vi "TDC_setHistogramParams.vi"(8 "Error In":errorcluster, 10 "Bin Count":i32, 11 "Bin Width":i32) -> (0 "Error Out":errorcluster)   [LabVIEW 2011]
uses:
  tdcbase.dll
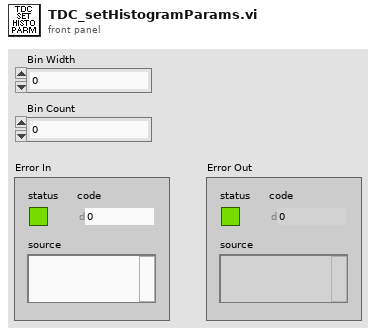
[diagram p1: front panel]
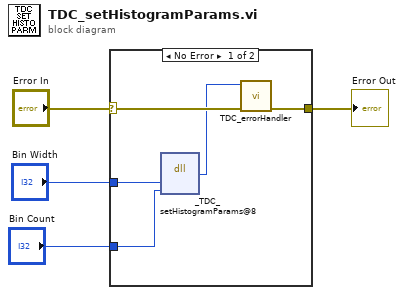
[diagram p0: block diagram]
diagram:
  n1 = case shown="No Error" "Error In" {
    selector: "Error In" -> [w9 w10]
    tunnel: [w8 w10] -> w3
    tunnel: "Bin Width" -> [w6 _]
    tunnel: "Bin Count" -> [w5 _]
    frame No Error {
      n2 = dll-call lib="X:/tdcbase.dll" fn="_TDC_setHistogramParams@8"("binWidth"=w6, "binCount"=w5) -> ("return type"=w7:i32)  [unwired: 5 in, 2 out]
      n3 = call "TDC_errorHandler.vi"("Error In"=w9, "TDC Return Code"=w7) -> ("Error Out"=w8:errorcluster)  [unwired: 9 in]
    }
    frame Error {
    }
  }
  "Error Out" <- w3
